vi "ATWriteErd.vi"(0 "GEA2 Reference In":refnum<k24>, 5 "Destination":string, 7 "Erd Number":string, 9 "Data to write":string, 11 "Error In":errorcluster) -> (4 "GEA2 Reference Out":refnum<k24>, 15 "Error Out":errorcluster)   [LabVIEW 2021]
uses:
  D:/Common/LabVIEW GEA2 Toolkit/source/GEA3 DLL Source/GeaCommunication.dll
  Common/LabVIEW GEA2 Toolkit/source/GEA3 DLL Source/GeaCommunication.dll
  Common/LabVIEW GEA2 Toolkit/GEA3/type defs/ERD Write Data In.ctl
  Common/LabVIEW GEA2 Toolkit/GEA3/type defs/Data Type.ctl
  Common/LabVIEW GEA2 Toolkit/GEA3/library/GEA2_Toolkit.lvlib
panel:
  out "Raw Data Out":string[](array[string])
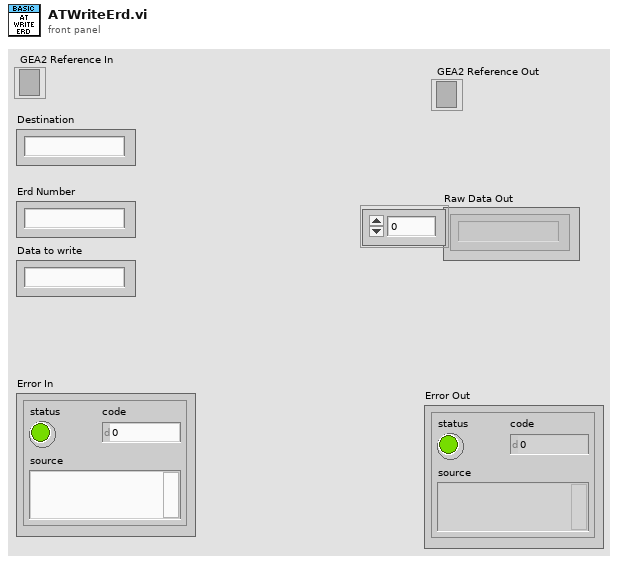
[diagram p1: front panel]
types:
  T1 = typedef "ERD Write Data In.ctl" = cluster{"ERD Number":u16, "Data Type":T2, "Data":string}
  T2 = typedef "Data Type.ctl" = enum16{"string", "boolean", "uint8_t", "uint16_t", "uint32_t", "uint64_t", "int8_t", "int16_t", "int32_t", "int64_t"}
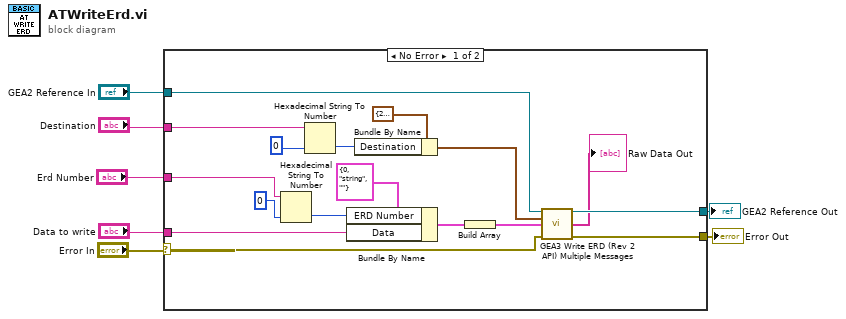
[diagram p0: block diagram]
diagram:
  n1 = case shown="No Error" "Error In" {
    selector: "Error In" -> [w10 w26]
    tunnel: "Destination" -> [w15 _]
    tunnel: "Data to write" -> [w14 _]
    tunnel: [w13 w25] -> w5
    tunnel: [w12 w26] -> w4
    tunnel: "GEA2 Reference In" -> [w11 w25]
    tunnel: "Erd Number" -> [w9 _]
    frame No Error {
      n2 = Hexadecimal String To Number(string=w9, default (0uL)=u16 0 ("ERD Number")) -> (number=w18:u16)  [unwired: 1 in, 1 out]
      n3 = Hexadecimal String To Number(string=w15, default (0uL)=u8 0 ("Destination")) -> (number=w23:u8)  [unwired: 1 in, 1 out]
      n4 = Bundle By Name(cluster=T1 {"ERD Number"=0, "Data Type"=enum."string", "Data"=""} ("ERD Write Data In"), "ERD Number"=w18, "Data"=w14) -> (w22:T1)
      n5 = Bundle By Name(cluster=cluster{"Source":u8, "Destination":u8} {"Source"=229, "Destination"=0} ("GEA Inputs"), "Destination"=w23) -> (w16:cluster{"Source":u8, "Destination":u8})
      n6 = Build Array(w22) -> (w17:T1[])
      n7 = call "GEA3 Write ERD (Rev 2 API) Multiple Messages.vi"("GEA2 Reference In"=w11, "GEA Inputs"=w16, "Write ERD List"=w17, "Error In"=w10) -> ("GEA2 Reference Out"=w13:refnum<k24>, "Raw Data Out"=→"Raw Data Out":string[], "Error Out"=w12:errorcluster)  [unwired: 9 in]
    }
    frame Error {
    }
  }
  "GEA2 Reference Out" <- w5
  "Error Out" <- w4
